vi "Configure Trigger.vi"(8 "error in":errorcluster, 11 "Scope PXI Base CFG in":refnum<class "Scope PXI Base CFG.lvclass">) -> (0 "error out":errorcluster, 3 "Scope PXI Base CFG out":refnum<class "Scope PXI Base CFG.lvclass">)   [LabVIEW 2023, in "Scope PXI Base CFG.lvclass"]
uses:
  Scope PXI Base CFG.lvclass
  <instrlib>/niScope/Controls/niScope trigger slope.ctl
  <instrlib>/niScope/Controls/niScope trigger source digital.ctl
  Configuration/Configuration JSON/Configuration JSON Base/CFG JSON.lvclass/CFG JSON.ctl
  Scope PXI Base CFG.lvclass/Scope PXI Base CFG.ctl
  49d2c016-646b-4808-92bd-86f31724cd2e.vi
  <vilib>/JDP Science/JSONtext/Find Item.vi
  <vilib>/JDP Science/JSONtext/Next JSON Value.vi
  <vilib>/JDP Science/JSONtext/String Subset.vi
  <vilib>/JDP Science/JSONtext/Parsing/Advance past next JSON Value (inlined COPY).vi
  <vilib>/JDP Science/JSONtext/Parsing/Advance past whitespace.vi
  <vilib>/JDP Science/JSONtext/Parsing/Advance past String.vi
  <vilib>/JDP Science/JSONtext/Parsing/Advance past Number.vi
  <vilib>/JDP Science/JSONtext/Parsing/Advance past Line Ending.vi
  <vilib>/JDP Science/JSONtext/Parsing/Parse Full Path or Item Name.vi
  <vilib>/JDP Science/JSONtext/Parsing/Advance past Array.vi
  <vilib>/JDP Science/JSONtext/Parsing/Advance past Object.vi
  <vilib>/JDP Science/JSONtext/support/Error Cluster From Code.vi
  <vilib>/JDP Science/JSONtext/Offset/Find Item Locations by Path.vi
  <vilib>/JDP Science/JSONtext/JSON text to Variant.vi
  <vilib>/Utility/error.llb/Error Cluster From Error Code.vi
  <instrlib>/niScope/Configure/Trigger/niScope Configure Trigger Edge.vi
  <instrlib>/niScope/Configure/Trigger/niScope Configure Trigger Digital.vi
  <instrlib>/niScope/Configure/Trigger/niScope Configure Trigger Immediate.vi
  <instrlib>/niScope/Configure/Trigger/niScope Configure Trigger Software.vi
  <vilib>/JDP Science/JSONtext/LVClass Serializer/JSONtext LVClass Serializer.lvclass
  <vilib>/ErrorRing/Error Ring.xnode
  Configuration/Configuration JSON/Configuration JSON Base/CFG JSON.lvclass
panel:
  out "trigger source":T1="VAL_RTSI_0" caption="trigger source (RTSI 0)"
  out "trigger slope":T2 items=["Positive", "Negative"]
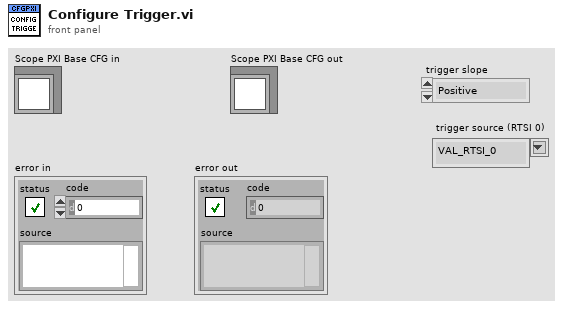
[diagram p1: front panel]
types:
  T1 = typedef "niScope trigger source digital.ctl" = string
  T2 = typedef "niScope trigger slope.ctl" = i32
  T3 = cluster{"Type":string, "Slope":string, "Source":string, "Holdoff":dbl, "Delay":dbl}
  T4 = typedef "LVStringsAndValuesArrayTypeDef_I32.ctl" = cluster{"String":string, "Value":i32}[]
  T5 = typedef "LVComboBoxStrsAndValuesArrayTypeDef.ctl" = cluster{"String":string, "Value":string}[]
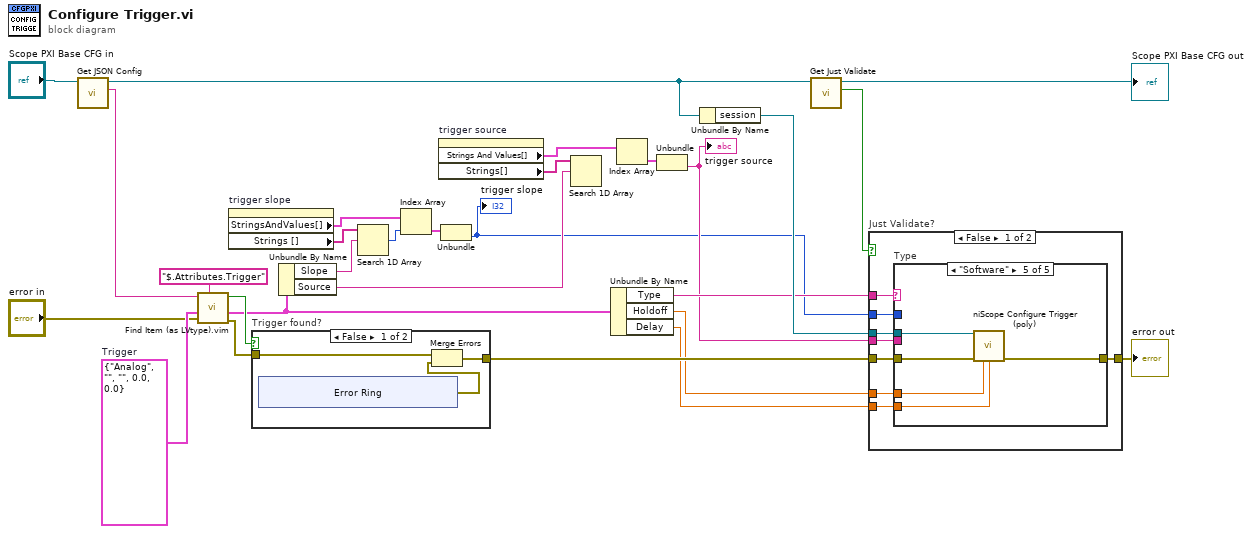
[diagram p0: block diagram]
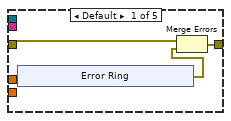
[diagram p2: hidden frame]
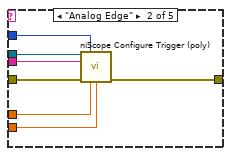
[diagram p3: hidden frame]
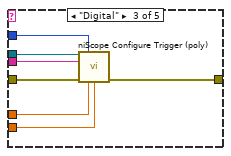
[diagram p4: hidden frame]
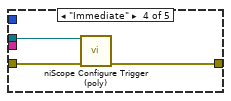
[diagram p5: hidden frame]
diagram:
  w16 = T3 {"Type"="Analog", "Slope"="", "Source"="", "Holdoff"=0.0, "Delay"=0.0}  # Trigger
  n1 = call "Get JSON Config.vi"("CFG Base in"="Scope PXI Base CFG in") -> ("<JSON>Config>"=w18:string, "CFG Base out"=w17:refnum<class "Scope PXI Base CFG.lvclass">)  [unwired: 9 in]
  n2 = call "Find Item (as LVtype).vim"("$Path or Item Name"="$.Attributes.Trigger", "error in (no error)"="error in", "Data Type and Default Value"=w16, "JSON"=w18) -> ("error out"=w13:errorcluster, "Data"=w10:T3, "Found"=w14:bool)  [unwired: 4 in, 1 out]
  n3 = property on="trigger slope" class="Ring (strict)"() -> ("StringsAndValues[]"=w24:T4, "Strings []"=w26:string[])  [unwired: 2 in, 2 out]
  n4 = case "Trigger found?" shown="False" w14 {
    tunnel: [w31 w37] -> w6
    tunnel: w13 -> [w29 w37]
    frame False {
      n5 = xnode "Error Ring"() -> ("error out"=w30:errorcluster)
      n6 = Merge Errors(w29, w30) -> (w31:errorcluster)
    }
    frame True {
    }
  }
  n7 = Unbundle By Name(w10) -> ("Slope"=w12:string, "Source"=w11:string)
  n8 = Search 1D Array(1D array=w26, element=w12) -> (index of element=w25:i32)  [unwired: 1 in]
  n9 = Index Array(array=w24, index=w25) -> (element=w23:cluster{"String":string, "Value":i32})
  n10 = property on="trigger source" class="CmbBox (strict)"() -> ("Strings And Values[]"=w22:T5, "Strings[]"=w15:string[])  [unwired: 2 in, 2 out]
  n11 = Unbundle(w23) -> ("Value"=w7:i32)  [unwired: 1 out]
  "trigger slope" <- w7
  n12 = Search 1D Array(1D array=w15, element=w11) -> ()  [unwired: 1 in, 1 out]
  n13 = Unbundle By Name(w10) -> ("Type"=w9:string, "Holdoff"=w4:dbl, "Delay"=w5:dbl)
  n14 = Index Array(array=w22) -> (element=w21:cluster{"String":string, "Value":string})  [unwired: 1 in]
  n15 = Unbundle(w21) -> ("Value"=w8:string)  [unwired: 1 out]
  "trigger source" <- w8
  n16 = Unbundle By Name(w17) -> ("session"=w20:refnum<k15>)
  n17 = call "Get Just Validate.vi"("CFG JSON Base in"=w17) -> ("Just Validate"=w2:bool, "CFG JSON Base out"=→"Scope PXI Base CFG out":refnum<class "Scope PXI Base CFG.lvclass">)  [unwired: 9 in]
  n18 = case "Just Validate?" shown="False" w2 {
    tunnel: [w45 w76] -> w27
    tunnel: w20 -> [w44 _]
    tunnel: w9 -> [w43 _]
    tunnel: w8 -> [w42 _]
    tunnel: w7 -> [w41 _]
    tunnel: w6 -> [w40 w76]
    tunnel: w5 -> [w39 _]
    tunnel: w4 -> [w38 _]
    frame False {
      n19 = case "Type" shown="\"Software\"" w43 {
        tunnel: w44 -> [_ w59 w66 w69 w75]
        tunnel: [w48 w60 w67 w70 w74] -> w45
        tunnel: w42 -> [_ w58 w64 _ _]
        tunnel: w41 -> [_ w57 w63 _ _]
        tunnel: w40 -> [w46 w56 w65 w68 w73]
        tunnel: w38 -> [_ w55 w62 _ w72]
        tunnel: w39 -> [_ w54 w61 _ w71]
        frame Default {
          n20 = xnode "Error Ring"() -> ("error out"=w47:errorcluster)
          n21 = Merge Errors(w46, w47) -> (w48:errorcluster)
        }
        frame "Analog Edge" {
          n22 = call-poly <instrlib>:"niScope Configure Trigger (poly).vi"("instrument handle"=w59, "trigger slope"=w57, "trigger source"=w58, "error in"=w56, "trigger holdoff"=w55, "trigger delay"=w54) -> ("error out"=w60:errorcluster)  [unwired: 8 in, 1 out]
        }
        frame "Digital" {
          n23 = call-poly <instrlib>:"niScope Configure Trigger (poly).vi"("instrument handle"=w66, "trigger slope"=w63, "trigger source"=w64, "error in"=w65, "trigger holdoff"=w62, "trigger delay"=w61) -> ("error out"=w67:errorcluster)  [unwired: 8 in, 1 out]
        }
        frame "Immediate" {
          n24 = call-poly <instrlib>:"niScope Configure Trigger (poly).vi"("instrument handle"=w69, "error in"=w68) -> ("error out"=w70:errorcluster)  [unwired: 12 in, 1 out]
        }
        frame "Software" {
          n25 = call-poly <instrlib>:"niScope Configure Trigger (poly).vi"("instrument handle"=w75, "error in"=w73, "trigger holdoff"=w72, "trigger delay"=w71) -> ("error out"=w74:errorcluster)  [unwired: 10 in, 1 out]
        }
      }
    }
    frame True {
    }
  }
  "error out" <- w27
